vi "Read Gain Limits(Log).vi"(8 "error in (no error)":errorcluster, 11 "APDClass in":refnum<class "APDClass.lvclass">) -> (0 "error out":errorcluster, 2 "GainLimits(Log)":cluster{"GainMax":dbl, "GainMin":dbl}, 3 "APDClass out":refnum<class "APDClass.lvclass">)   [LabVIEW 2020, in "APDClass.lvclass"]
uses:
  APDClass.lvclass
  APDClass.lvclass/APDClass.ctl
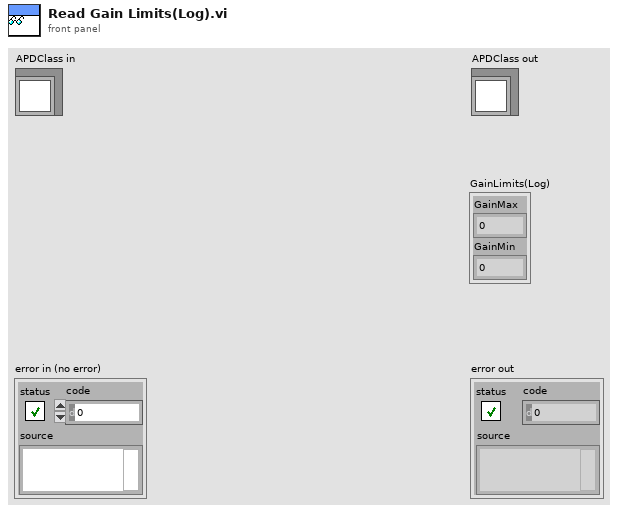
[diagram p1: front panel]
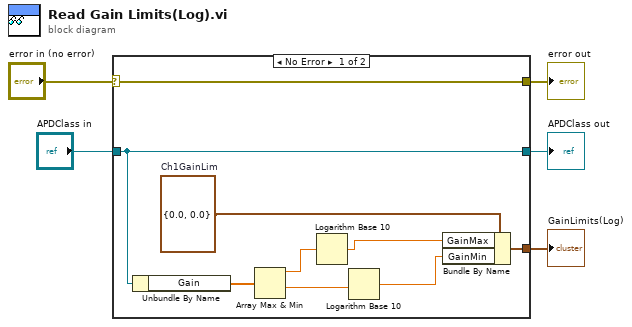
[diagram p0: block diagram]
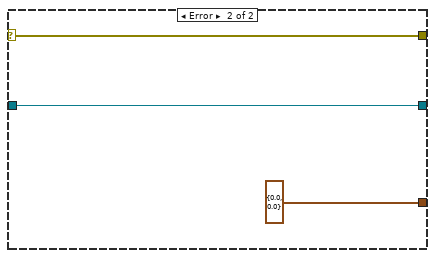
[diagram p2: hidden frame]
diagram:
  n1 = case shown="No Error" "error in (no error)" {
    selector: "error in (no error)" -> [w14 w16]
    tunnel: [w14 w16] -> w4
    tunnel: [w13 w17] -> w2
    tunnel: "APDClass in" -> [w13 w17]
    tunnel: [w11 cluster{"GainMin":dbl, "GainMax":dbl} {"GainMin"=0.0, "GainMax"=0.0} ("GainMinMax")] -> w1
    frame No Error {
      w10 = cluster{"GainMax":dbl, "GainMin":dbl} {"GainMax"=0.0, "GainMin"=0.0}  # Ch1GainLim
      n2 = Unbundle By Name(w13) -> ("Gain"=w12:dbl[])
      n3 = Array Max & Min(array=w12) -> (max value=w9:dbl, min value=w7:dbl)  [unwired: 2 out]
      n4 = Logarithm Base 10(1:w9) -> (0:w8:dbl)
      n5 = Logarithm Base 10(1:w7) -> (0:w6:dbl)
      n6 = Bundle By Name(cluster=w10, "GainMax"=w8, "GainMin"=w6) -> (w11:cluster{"GainMax":dbl, "GainMin":dbl})
    }
    frame Error {
    }
  }
  "error out" <- w4
  "APDClass out" <- w2
  "GainLimits(Log)" <- w1
